vi "Calibrate Zero.vi"(8 "error in (no error)":errorcluster, 9 "Steps from ZERO":i32 min=-32767 step=1, 10 "MONO. NUMBER\n(DK242 only)":u8=1 min=1 max=2 step=1, 11 "VISA resource name":refnum<visa-resource-name>) -> (0 "error out":errorcluster, 3 "VISA resource name out":refnum<visa-resource-name>)   [LabVIEW 2009, in "Digikrom DK24x.lvlib"]
doc: "This command sets the current wavelength to 0.00nm.\n\nCAUTION: Use of this command will erase factory settings."
uses:
  Digikrom DK24x.lvlib
  Private/Command.ctl
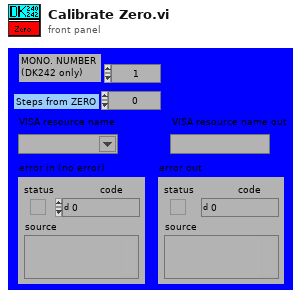
[diagram p1: front panel]
types:
  T1 = typedef "Digikrom DK24x.lvlib/Command.ctl" = u8
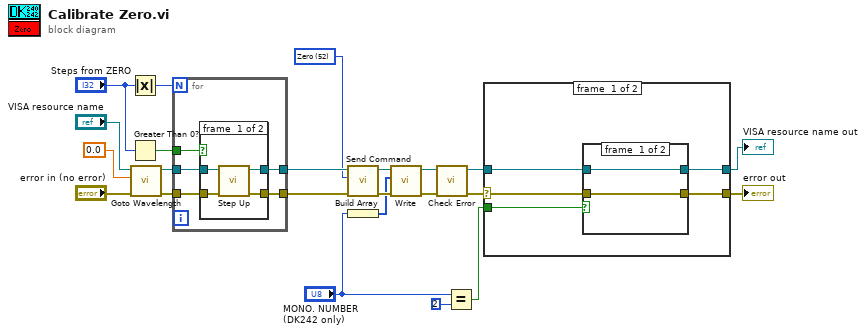
[diagram p0: block diagram]
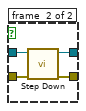
[diagram p2: hidden frame]
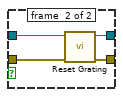
[diagram p3: hidden frame]
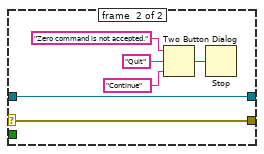
[diagram p4: hidden frame]
diagram:
  w1 = T1 52 items=["Cancel"=24, "Clear"=25, "CSR"=28, "Echo"=27, "Filter"=15, "Gcal"=18, "Goto"=16, "Grtid?"=19, "Grtsel"=26, "NOVRAM Read"=56, "NOVRAM Write"=59, "Reset"=255, "Scan"=12, "Scan Up"=9, "Scan Down"=3, "Serial?"=33, "Slew Up"=8, "Slew Down"=2, "Slit Reset"=43, "Slit?"=30, "Sltadj"=14, "Speed"=13, "Sspeed?"=21, "Step Down"=1, "Step Up"=7, "S1adj"=31, "S2adj"=32, "S3adj"=34, "S1cal"=22, "S2cal"=23, "S3cal"=35, "Test"=17, "Type"=57, "Wave?"=29, "Zero"=52] ("Command")
  n1 = Absolute Value(x="Steps from ZERO") -> (abs(x)=w12:i32)
  n2 = Greater Than 0?(x="Steps from ZERO") -> (x > 0?=w7:bool)
  n3 = call "Goto Wavelength.vi"("error in (no error)"="error in (no error)", "WAVELENGTH"=dbl[unit] 0.0, "VISA resource name"="VISA resource name") -> ("error out"=w20:errorcluster, "VISA resource name out"=w21:refnum<visa-resource-name>)  [unwired: 7 out]
  n4 = for {
    N: w12 -> [_]
    tunnel: w7 -> [w24]
    tunnel: w21 -> [w27]
    tunnel: [w25] -> w14
    tunnel: w20 -> [w28]
    tunnel: [w26] -> w15
    n5 = case shown="True" w24 {
      tunnel: w28 -> [w32 w36]
      tunnel: w27 -> [w31 w35]
      tunnel: [w29 w34] -> w26
      tunnel: [w30 w33] -> w25
      frame #0 {
        n6 = call "Step Up.vi"("error in (no error)"=w32, "VISA resource name"=w31) -> ("error out"=w29:errorcluster, "VISA resource name out"=w30:refnum<visa-resource-name>)  [unwired: 8 out]
      }
      frame #1 {
        n7 = call "Step Down.vi"("error in (no error)"=w36, "VISA resource name"=w35) -> ("error out"=w34:errorcluster, "VISA resource name out"=w33:refnum<visa-resource-name>)  [unwired: 6 out]
      }
    }
  }
  n8 = call "Send Command.vi"("error in (no error)"=w15, "Command"=w1, "VISA resource name"=w14) -> ("error out"=w17:errorcluster, "VISA resource name out"=w16:refnum<visa-resource-name>)  [unwired: 7 out]
  n9 = Build Array("MONO. NUMBER\n(DK242 only)") -> (w2:u8[])
  n10 = call "Write.vi"("error in (no error)"=w17, "Byte Array"=w2, "VISA resource name"=w16) -> ("error out"=w11:errorcluster, "VISA resource name out"=w10:refnum<visa-resource-name>)  [unwired: 7 out]
  n11 = call "Check Error.vi"("error in"=w11, "VISA resource name in"=w10) -> ("error out"=w19:errorcluster, "VISA resource name out"=w18:refnum<visa-resource-name>)  [unwired: 1 in, 7 out]
  n12 = Equal?(x="MONO. NUMBER\n(DK242 only)", y=u8 2) -> (x = y?=w8:bool)
  n13 = case shown="No Error" w19 {
    selector: w19 -> [w40 w53]
    tunnel: w8 -> [w41 _]
    tunnel: w18 -> [w39 w52]
    tunnel: [w38 w52] -> w6
    tunnel: [w37 w53] -> w5
    frame #0 {
      n14 = case shown="True" w41 {
        tunnel: w40 -> [w43 w46]
        tunnel: w39 -> [w42 w47]
        tunnel: [w42 w45] -> w38
        tunnel: [w43 w44] -> w37
        frame #0 {
        }
        frame #1 {
          n15 = call "Reset Grating.vi"("error in (no error)"=w46, "VISA resource name"=w47) -> ("error out"=w44:errorcluster, "VISA resource name out"=w45:refnum<visa-resource-name>)  [unwired: 8 out]
        }
      }
    }
    frame #1 {
      n16 = Two Button Dialog(message="Zero command is not accepted.", 1:"Continue", 2:"Quit") -> (T button?=w48:bool)
      n17 = Stop(stop? (T)=w48) -> ()
    }
  }
  "error out" <- w5
  "VISA resource name out" <- w6
